vi "Read Auto Text File.vi"(8 "error in":errorcluster, 11 "selected path":path) -> (0 "error out":errorcluster, 2 "Programs":string[](array[string]), 3 "Program Name":string[](array[string]))   [LabVIEW 2013]
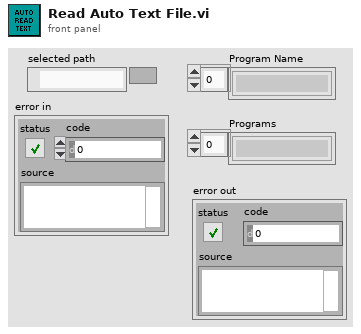
[diagram p1: front panel]
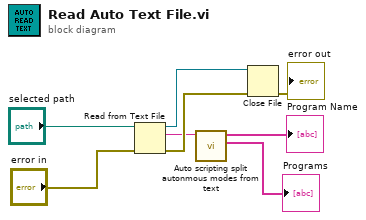
[diagram p0: block diagram]
diagram:
  n1 = Read from Text File(file (use dialog)="selected path", error in="error in") -> (refnum out=w7:refnum<file>, text=w3:string, error out=w8:errorcluster)  [unwired: 2 in, 1 out]
  n2 = call "Auto scripting split autonmous modes from text.vi"("String"=w3) -> ("Programs"=→"Programs":string[], "Program Name"=→"Program Name":string[])  [unwired: 9 in]
  n3 = Close File(refnum=w7, error in=w8) -> (error out=→"error out":errorcluster)  [unwired: 1 out]
